vi "Converter - Data Array to Binary.vi"(1 "Data bit array":bool[](array[boolean])=[FALSE, FALSE, FALSE, FALSE, FALSE, FALSE, FALSE, FALSE]) -> (0 "Value":u32 format="%b")   [LabVIEW 2013]
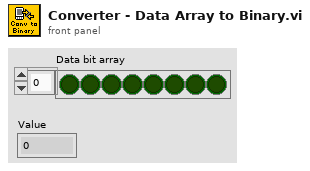
[diagram p1: front panel]
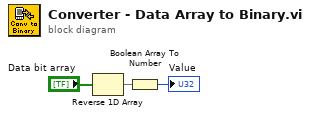
[diagram p0: block diagram]
diagram:
  n1 = Reverse 1D Array(array="Data bit array") -> (reversed array=w2:bool[])
  n2 = Boolean Array To Number(Boolean array=w2) -> (number=→"Value":u8)
